vi "Calculate Number of Text Rows.vi"(0 "Library Path":path, 5 "Number of Pixel Rows in Icon":i32) -> (4 "Number of Text Rows":i32)   [LabVIEW 2020, in "Text-Based VI Icon.lvlib"]
uses:
  <vilib>/LabVIEW Icon API/Set Text Icon/Text-Based VI Icon.lvlib
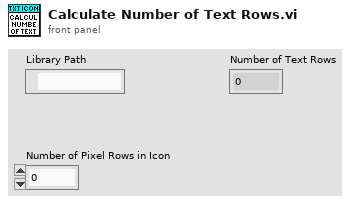
[diagram p1: front panel]
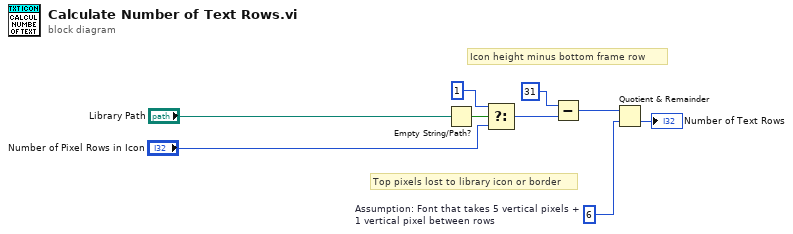
[diagram p0: block diagram]
diagram:
  w9 = 6  # Assumption: Font that takes 5 vertical pixels + 1 vertical pixel between rows
  # "Icon height minus bottom frame row"
  # "Top pixels lost to library icon or border"
  n1 = Empty String/Path?(string/path="Library Path") -> (empty?=w6:bool)
  n2 = Select(t=1, s=w6, f="Number of Pixel Rows in Icon") -> (s? t:f=w2:i32)
  n3 = Subtract(x=31 ("t"), y=w2) -> (x-y=w1:i32)
  n4 = Quotient & Remainder(x=w1, y=w9) -> (floor(x/y)=→"Number of Text Rows":i32)  [unwired: 1 out]
